vi "read-write config ini.vi"   [LabVIEW 2024]
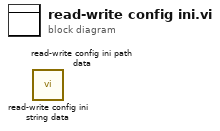
[diagram p0: block diagram]
diagram:
  n1 = call "read-write config ini string data.vi"() -> ()  [unwired: 10 in, 2 out]
  n2 = call "read-write config ini path data.vi"() -> ()  [unwired: 10 in, 2 out]
